vi "Elliptic IIR Filter Design.vi"() -> ()   [LabVIEW 2023]
doc: "Demonstrates how to use the Advanced FIR Filter Design VIs and the Advanced IIR Filter Design VIs to design filters with a specified filter order or an estimated filter order. This example uses the DFD Elliptic Order Estimation VI and the DFD Elliptic Design VI to design an infinite impulse response (IIR) filter using the Elliptic method. The LabVIEW Digital Filter Design Toolkit provides order estimation and design VIs for other design methods, such as Dolph-Chebyshev Window, Kaise Window, Bessel, etc..\n\nComplete the following steps to use this VI.\n1) Run the VI.\n2) Change the filter specifications and filter order on the <B>Specified Order</B> page.\n3) Observe the magnitude response and phase response, which might not meet the specifications if the filter order is too low.\n4) Verify if the <B>Actual Filter Order</B> equals the filter order you specified.\n5) View the <B>Estimated Order</B> page and change the specifications.\n6) Observe the magnitude response, phase response, and actual filter order.\n7) Click the <B>STOP</B> button to stop this VI.\n8) Examine the block diagram to learn how to design a filter with an automatically estimated filter order."
uses:
  <vilib>/addons/Digital Filter Design/_Objects.llb/DFD Filter Frequence Specification (Design).ctl
  <vilib>/addons/Digital Filter Design/_Objects.llb/DFD Filter Ripple Specification (Design).ctl
  <vilib>/addons/Digital Filter Design/_Objects.llb/DFD Phase Setting.ctl
  <vilib>/addons/Digital Filter Design/Analysis.llb/DFD Plot Freq Response (Linear-Spaced).vi
  <vilib>/addons/Digital Filter Design/NI_DigFilterLicensed.lvlib
panel:
  out "Actual Filter Order":i32
  in  "Sampling Frequency [Hz]":dbl=1000.0 format="%.2f"
  out "Error Message":string
  in  "stop":bool
  out "Phase Response":cluster{"f0":dbl, "df":dbl, "values":dbl[]}[](graph)
  out "Magnitude Response":cluster{"f0":dbl, "df":dbl, "values":dbl[]}[](graph)
  in  "Filter Order Sel":enum32{"Specified Order", "Estimated Order"}(tab)
  in  "Filter Type":u16(ring)=2 items=["Lowpass", "Highpass", "Bandpass", "Bandstop"]
  in  "Ripples [dB]":T1={"passband ripple"=0.1, "stopband atten"=60.0} {"stopband atten" format="%.2f"; "passband ripple" format="%.2f"}
  in  "High Cutoff Frequency [Hz]":dbl=350.0
  in  "Low Cutoff Frequency [Hz]":dbl=250.0
  in  "Order":i32=8
  in  "Ripple Specifications":T2={"passband"=0.1, "stopband"=60.0, "dB/linear? (T: dB)"=TRUE}
  in  "Frequency Sepcifications [Hz]":T3={"fpass 1"=250.0, "fstop 1"=150.0, "fpass 2 "=350.0, "fstop 2"=450.0}
  in  "Filter Type":u16(ring)=2 items=["Lowpass", "Highpass", "Bandpass", "Bandstop"]
  # "Select Help>>Show Context Help and move the cursor over the VI icon for more information."
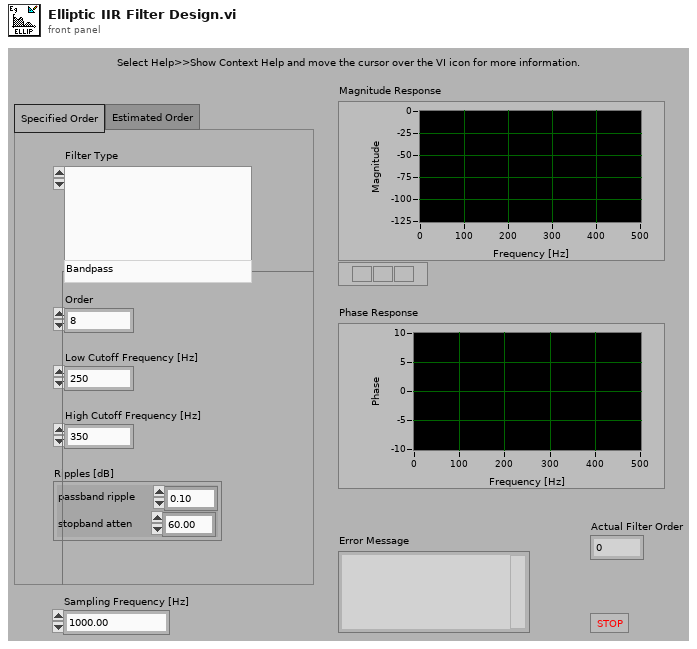
[diagram p1: front panel]
types:
  T1 = cluster{"passband ripple":dbl, "stopband atten":dbl}
  T2 = typedef "NI_DigFilterLicensed.lvlib/DFD Filter Ripple Specification (Design).ctl" = cluster{"passband":dbl, "stopband":dbl, "dB/linear? (T: dB)":bool}
  T3 = typedef "NI_DigFilterLicensed.lvlib/DFD Filter Frequence Specification (Design).ctl" = cluster{"fpass 1":dbl, "fstop 1":dbl, "fpass 2 ":dbl, "fstop 2":dbl}
  T4 = typedef "NI_DigFilterLicensed.lvlib/DFD Phase Setting.ctl" = cluster{"unwrap? (F)":bool, "degree? (F)":bool}
  T5 = typedef "NI_DigFilterLicensed.lvlib/DFD Filter Obj.ctl" = cluster{"mSRate_Fs":dbl, "mSRate_Version":string, "mSRate_Comments":string, "mSRate_OrgCoef":T6, "mSRate_CurCoef":T6, "mSRate_Quantized?":bool, "mSRate_QCoef":T6, "mSRate_QSettings":T8[], "mSRate_Order":i32, "mSRate_Scaling":cluster{"mSRate_ScaleByPowerOf2?":bool, "mSRate_ScaleType":T10}}
  T6 = typedef "NI_DigFilterLicensed.lvlib/DFD Filter Coef.ctl" = cluster{"type":T7, "gain":dbl, "coef a (k)":dbl[], "coef b (v)":dbl[]}
  T7 = typedef "NI_DigFilterLicensed.lvlib/DFD Filter Structure Type Selector.ctl" = enum16{"Undefined", "FIR Direct Form", "FIR Direct Form Transposed", "FIR Symmetric", "FIR Antisymmetric", "IIR Direct Form I", "IIR Direct Form I Transposed", "IIR Direct Form II", "IIR Direct Form II Transposed", "IIR Cascaded Second Order Sections Form I", "IIR Cascaded Second Order Sections Form I Transposed", "IIR Cascaded Second Order Sections Form II", "IIR Cascaded Second Order Sections Form II Transposed", "Lattice Allpass (basic sections)", "Lattice Allpass (one multiplier sections)", "Lattice Allpass (normalized sections)", "Lattice AR (basic sections)", "Lattice AR (one multiplier sections)", "Lattice AR (normalized sections)", "Lattice MA (minimum phase)", "Lattice MA (maximum phase)", "Lattice ARMA (basic sections)", "Lattice ARMA (one multiplier sections)", "Lattice ARMA (normalized sections)"}
  T8 = typedef "NI_DigFilterLicensed.lvlib/dfd_Internal Quantization Settings.ctl" = cluster{"source":T9, "wl":i16, "iwl":i16, "overflow mode":enum16{"Saturation", "Wrap"}, "rounding mode":enum16{"Nearest", "Truncation"}, "signed?":bool}
  T9 = typedef "NI_DigFilterLicensed.lvlib/dfd_Internal Quantization Srcs.ctl" = u16
  T10 = typedef "NI_DigFilterLicensed.lvlib/DFD Coef Norm Type.ctl" = enum16{"No Norm", "Time Domain 1-Norm", "Time Domain 2-Norm", "Time Domain Inf-Norm"}
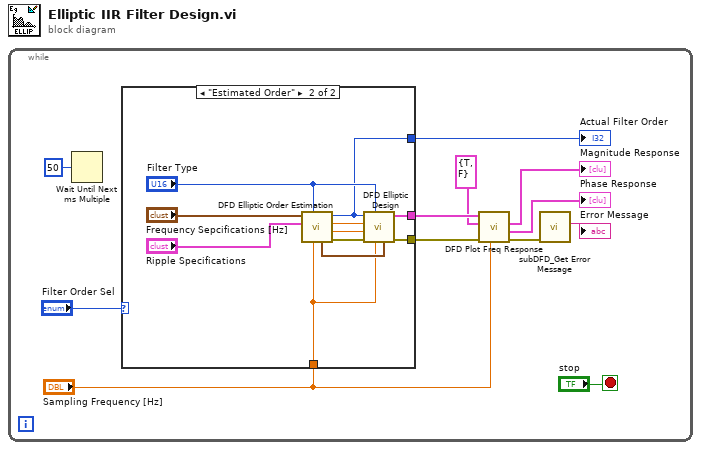
[diagram p0: block diagram]
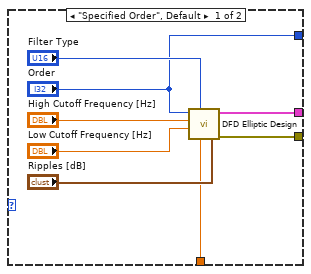
[diagram p2: hidden frame]
diagram:
  n1 = while {
    stop <- "stop" stop-if-true
    n2 = Wait Until Next ms Multiple(millisecond multiple=u32 50) -> ()  [unwired: 1 out]
    n3 = case shown="\"Estimated Order\"" "Filter Order Sel" {
      tunnel: [w18 w31] -> w7
      tunnel: "Sampling Frequency [Hz]" -> [w16 w23]
      tunnel: [w15 w30] -> w6
      tunnel: ["Order" w22] -> w10
      frame "Specified Order", Default {
        n4 = call <vilib>:"DFD Elliptic Design.vi"("ripples [dB]"="Ripples [dB]", "fs [Hz]"=w16, "filter type"="Filter Type", "low cutoff freq [Hz]"="Low Cutoff Frequency [Hz]", "high cutoff freq [Hz]"="High Cutoff Frequency [Hz]", "order"="Order") -> ("error out"=w15:errorcluster, "filter out"=w18:T5)  [unwired: 1 in, 3 out]
      }
      frame "Estimated Order" {
        n5 = call <vilib>:"DFD Elliptic Order Estimation.vi"("fs [Hz]"=w23, "filter type"="Filter Type", "ripple specs"="Ripple Specifications", "freq specs [Hz]"="Frequency Sepcifications [Hz]") -> ("error out"=w29:errorcluster, "low cutoff freq [Hz]"=w27:dbl, "high cutoff freq [Hz]"=w28:dbl, "estimated order"=w22:i32, "ripples [dB]"=w26:T1)  [unwired: 1 in, 2 out]
        n6 = call <vilib>:"DFD Elliptic Design.vi"("ripples [dB]"=w26, "fs [Hz]"=w23, "filter type"="Filter Type", "error in (no error)"=w29, "low cutoff freq [Hz]"=w27, "high cutoff freq [Hz]"=w28, "order"=w22) -> ("error out"=w30:errorcluster, "filter out"=w31:T5)  [unwired: 3 out]
      }
    }
    "Actual Filter Order" <- w10
    n7 = call-poly <vilib>:"DFD Plot Freq Response.vi"("fs [Hz]"="Sampling Frequency [Hz]", "error in (no error)"=w6, "phase view"=T4 {"unwrap? (F)"=TRUE, "degree? (F)"=FALSE}, "filter in"=w7) -> ("error out"=w2:errorcluster, "phase response"=→"Phase Response":cluster{"f0":dbl, "df":dbl, "values":dbl[]}[], "magnitude response"=→"Magnitude Response":cluster{"f0":dbl, "df":dbl, "values":dbl[]}[])  [unwired: 4 in, 1 out]
    n8 = call <vilib>:"subDFD_Get Error Message.vi"("error in (no error)"=w2) -> ("Error Message"=→"Error Message":string)  [unwired: 10 out]
  }
